vi "Bridge Setup.vi"(8 "error in":errorcluster, 10 "sampling":T2, 11 "bridge in":T3) -> (0 "error out":errorcluster, 3 "bridge out":T3)   [LabVIEW 2013]
doc: "Setup bridge parameters."
uses:
  Bridge Session.ctl
  Bridge Type.ctl
  drivers/TWM client/TWM Session.ctl
  drivers/TWM client/TWM Mode.ctl
  Bridge Sampling Setup.ctl
  drivers/TWM client.lvlibp/TWM client/TWM Client Meas Setup.ctl
  drivers/TWM client.lvlibp/TWM client/TWM Client Processing Setup.ctl
  drivers/TWM client.lvlibp
panel:
  in  "TWM.mode":T1
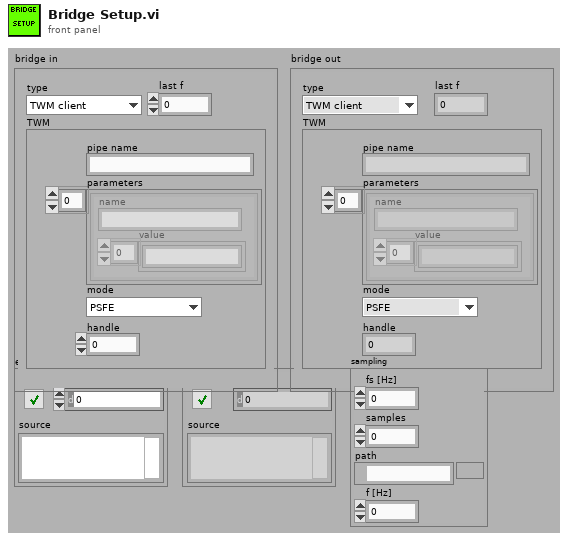
[diagram p1: front panel]
types:
  T1 = typedef "TWM Mode.ctl" = enum16{"PSFE", "FPNLSF", "FFT"}
  T2 = typedef "Bridge Sampling Setup.ctl" = cluster{"fs [Hz]":dbl, "samples":i32, "path":path, "f [Hz]":dbl}
  T3 = typedef "Bridge Session.ctl" = cluster{"type":T4, "TWM":T5, "last f":dbl}
  T4 = typedef "Bridge Type.ctl" = enum16{"TWM client", "dummy"}
  T5 = typedef "TWM Session.ctl" = cluster{"pipe name":string, "parameters":cluster{"name":string, "value":string[]}[], "mode":T1, "handle":i32}
  T6 = typedef "TWM client.lvlibp/TWM Client Processing Setup.ctl" = cluster{"calculate":i32, "all cycles at once":bool, "alg. ID":string, "unc mode":string, "mc cycles":i32, "timeout [s]":dbl, "loc [-]":dbl, "valid?":bool, "qwtb params":cluster{"name":string, "data":string[]}[]}
  T7 = typedef "TWM client.lvlibp/TWM Client Meas Setup.ctl" = cluster{"smpl count":i32, "smpl rate [Hz]":dbl, "average":i32, "aperture [s]":dbl, "valid?":bool, "meas fld":path}
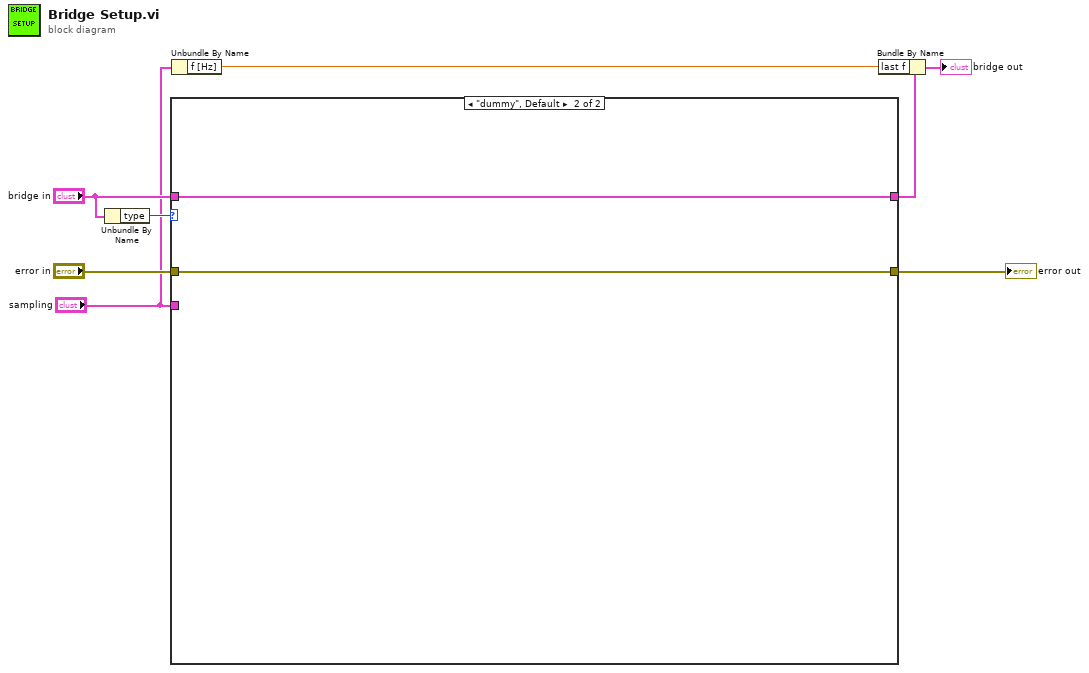
[diagram p0: block diagram]
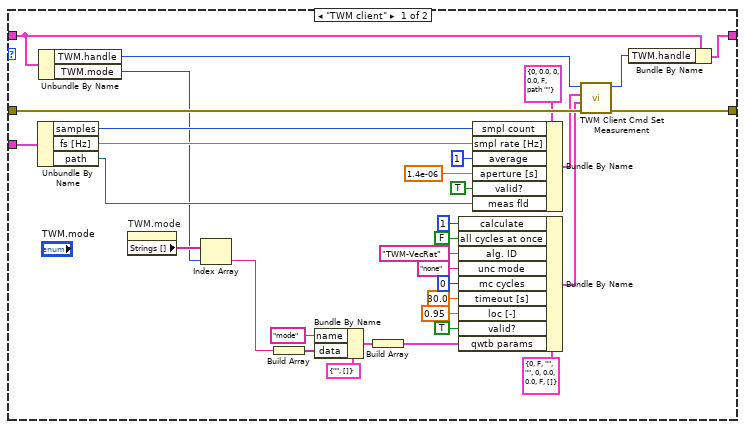
[diagram p2: hidden frame]
diagram:
  n1 = Unbundle By Name("bridge in") -> ("type"=w8:T4)
  n2 = case shown="\"dummy\", Default" w8 {
    tunnel: "error in" -> [w38 w43]
    tunnel: [w36 w43] -> w6
    tunnel: "bridge in" -> [w41 w42]
    tunnel: [w40 w42] -> w4
    tunnel: "sampling" -> [w33 _]
    frame "TWM client" {
      n3 = Unbundle By Name(w33) -> ("samples"=w20:i32, "fs [Hz]"=w19:dbl, "path"=w32:path)
      n4 = Unbundle By Name(w41) -> ("TWM.handle"=w39:i32, "TWM.mode"=w16:T1)
      n5 = property on="TWM.mode" class="Enum (strict)"() -> ("Strings []"=w17:string[])  [unwired: 2 in, 2 out]
      n6 = Index Array(array=w17, index=w16) -> (element=w13:string)
      n7 = Build Array(w13) -> (w14:string[])
      n8 = Bundle By Name(cluster=cluster{"name":string, "data":string[]} {"name"="", "data"=[]} ("Cluster"), "name"="mode", "data"=w14) -> (w11:cluster{"name":string, "data":string[]})
      n9 = Build Array(w11) -> (w10:cluster{"name":string, "data":string[]}[])
      n10 = Bundle By Name(cluster=T6 {"calculate"=0, "all cycles at once"=FALSE, "alg. ID"="", "unc mode"="", "mc cycles"=0, "timeout [s]"=0.0, "loc [-]"=0.0, "valid?"=FALSE, "qwtb params"=[]} ("processing"), "calculate"=1, "all cycles at once"=FALSE, "alg. ID"="TWM-VecRat", "unc mode"="none", "mc cycles"=0, "timeout [s]"=30.0, "loc [-]"=0.95, "valid?"=TRUE, "qwtb params"=w10) -> (w27:T6)
      n11 = Bundle By Name(cluster=T7 {"smpl count"=0, "smpl rate [Hz]"=0.0, "average"=0, "aperture [s]"=0.0, "valid?"=FALSE, "meas fld"=path ""} ("meas"), "smpl count"=w20, "smpl rate [Hz]"=w19, "average"=1, "aperture [s]"=1.4e-06, "valid?"=TRUE, "meas fld"=w32) -> (w34:T7)
      n12 = call "TWM Client Cmd Set Measurement.vi"("error in"=w38, "processing"=w27, "meas"=w34, "handle"=w39) -> ("error out"=w36:errorcluster, "handle out"=w37:i32)  [unwired: 6 in]
      n13 = Bundle By Name(cluster=w41, "TWM.handle"=w37) -> (w40:T3)
    }
    frame "dummy", Default {
    }
  }
  "error out" <- w6
  n14 = Unbundle By Name("sampling") -> ("f [Hz]"=w1:dbl)
  n15 = Bundle By Name(cluster=w4, "last f"=w1) -> (→"bridge out":T3)
